vi "Agilent PSG MXG Series Digital Modulation.vi"() -> ()   [LabVIEW 2018]
doc: "This example shows how to configure the I/Q modulator and dual arbitrary waveform generator.\n\n<b>Notes:</b>\n(1) This VI is valid only in E8267C, E8267D, N5162A, N5182A, N5172B, N5182B.\n(2) For E8267C, this VI is valid only when the instrument installs <B>Option 002</B> (Internal baseband generator) or <B>Option 602</B> (Digital bus baseband generator).\n(3) For E8267D, this VI is valid only when the instrument installs <B>Option 601</B> or <B>Option 602</B> (Internal baseband generator).\n(4) For N5162A and N5182A, this VI is valid only when the instrument installs <B>Option 651</B> or <B>Option 652</B> or <B>Option 654</B> (Internal baseband generator)."
uses:
  Agilent PSG MXG Series.lvlib
panel:
  in  "I/Q Source (0: Ext 50 Ohms)":u16(ring) items=["Ext 50 Ohms", "Ext 600 Ohms", "Internal", "Baseband Generator", "Off", "Sum"]
  in  "VISA resource name":refnum<visa-resource-name>
  in  "Enable ARB (T:Enable)":bool=TRUE
  in  "External Q Offset (50 mV)":dbl=0.05
  in  "External I Offset (50 mV)":dbl=0.05
  in  "Differential Mode Q Offset (10 mV)":dbl=0.01
  in  "Differential Mode I Offset (10 mV)":dbl=0.01
  in  "Common Mode I/Q Offset (1 V)":dbl=1.0
  in  "Q Offset (10 percent)":dbl=10.0
  in  "I/Q Skew (0 s)":dbl
  in  "Quadrature Skew (5 deg)":dbl=5.0
  in  "Gain (0.5 dB)":dbl=0.5
  in  "I Offset (10 percent)":dbl=10.0
  in  "Enable I/Q Adjustment (F:Disable)":bool
  in  "I/Q Source No. (1)":u16(ring)=1 items=["1"=1, "2"=2]
  in  "I/Q Phase Polarity (0: Normal)":u16(ring) items=["Normal", "Inverted"]
  # "(c) 2007-2016 National Instruments.  ALL RIGHTS RESERVED."
  # "(1) This VI is valid only in E8267C, E8267D, N5162A, N5182A, N5172B, N5182B.\n(2) For E8267C, this VI is valid only when the instrument installs Option 002 or Option 602.\n(3) For E8267D, this VI is valid only when the instrument installs Option 601 or Option 602.\n(4) For N5162A and N5182A, this VI is valid only when the instrument installs Option 651 or Option 652 or Option 654."
  # "Note: Enable arbitrary\nwaveform generator."
  # "Note: These parameters are\nfor I/Q Adjustment."
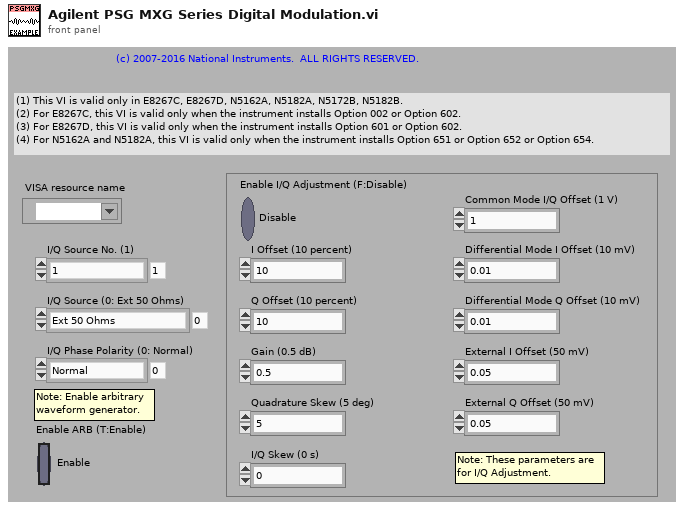
[diagram p1: front panel]
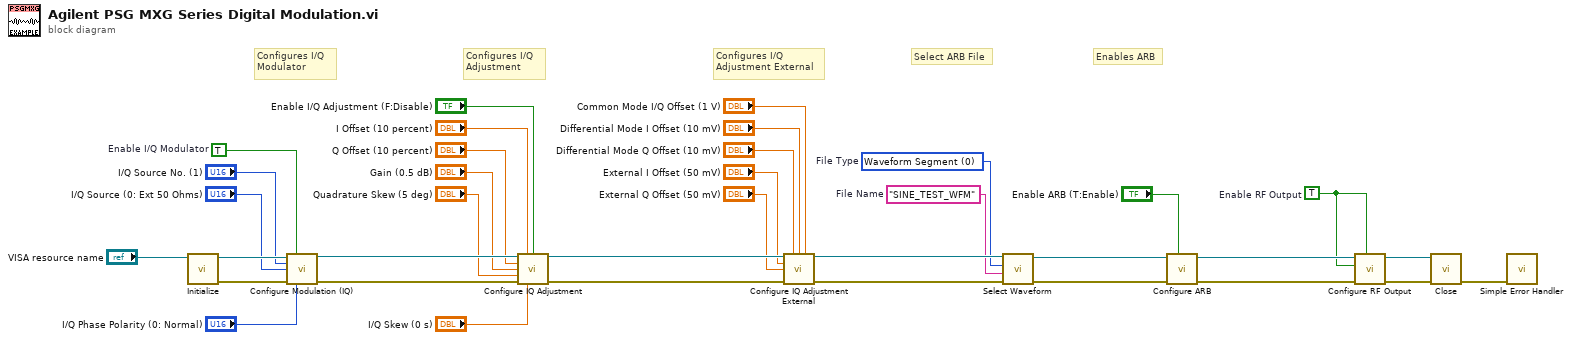
[diagram p0: block diagram]
diagram:
  w1 = TRUE  # Enable RF Output
  w11 = "SINE_TEST_WFM"  # File Name
  w12 = u16 0 items=["Waveform Segment", "Waveform Sequence"]  # File Type
  w33 = TRUE  # Enable I/Q Modulator
  # "Enables ARB"
  # "Select ARB File"
  # "Configures I/Q\nAdjustment External"
  # "Configures I/Q\nAdjustment"
  # "Configures I/Q\nModulator"
  n1 = call "Initialize.vi"("VISA resource name"="VISA resource name") -> ("error out"=w34:errorcluster, "VISA resource name out"=w35:refnum<visa-resource-name>)  [unwired: 3 in, 6 out]
  n2 = call "Configure Modulation (IQ).vi"("VISA resource name"=w35, "Enable I/Q Modulator (T:Enable)"=w33, "I/Q Source No. (1)"="I/Q Source No. (1)", "I/Q Source (0: Ext 50 Ohms)"="I/Q Source (0: Ext 50 Ohms)", "error in (no error)"=w34, "I/Q Phase Polarity (0: Normal)"="I/Q Phase Polarity (0: Normal)") -> ("VISA resource name out"=w30:refnum<visa-resource-name>, "error out"=w29:errorcluster)  [unwired: 4 in, 4 out]
  n3 = call "Configure IQ Adjustment.vi"("VISA resource name"=w30, "I Offset (0 percent)"="I Offset (10 percent)", "Enable I/Q Adjustment (F:Disable)"="Enable I/Q Adjustment (F:Disable)", "Q Offset (0 percent)"="Q Offset (10 percent)", "Gain (0 dB)"="Gain (0.5 dB)", "Quadrature Skew (0 deg)"="Quadrature Skew (5 deg)", "error in (no error)"=w29, "I/Q Skew (0 s)"="I/Q Skew (0 s)") -> ("VISA resource name out"=w22:refnum<visa-resource-name>, "error out"=w21:errorcluster)  [unwired: 2 in, 4 out]
  n4 = call "Configure IQ Adjustment External.vi"("VISA resource name"=w22, "Differential Mode Q Offset (0 V)"="Differential Mode Q Offset (10 mV)", "Differential Mode I Offset (0 V)"="Differential Mode I Offset (10 mV)", "Common Mode I/Q Offset (0 V)"="Common Mode I/Q Offset (1 V)", "External I Offset (0 V)"="External I Offset (50 mV)", "External Q Offset (0 V)"="External Q Offset (50 mV)", "error in (no error)"=w21) -> ("VISA resource name out"=w14:refnum<visa-resource-name>, "error out"=w13:errorcluster)  [unwired: 3 in, 4 out]
  n5 = call "Select Waveform.vi"("error in (no error)"=w13, "File Name (\"\")"=w11, "File Type (0: Waveform Segment)"=w12, "VISA resource name"=w14) -> ("error out"=w9:errorcluster, "VISA resource name out"=w10:refnum<visa-resource-name>)  [unwired: 6 out]
  n6 = call "Configure ARB.vi"("Enable ARB (T:Enable)"="Enable ARB (T:Enable)", "error in (no error)"=w9, "VISA resource name"=w10) -> ("error out"=w4:errorcluster, "VISA resource name out"=w5:refnum<visa-resource-name>)  [unwired: 1 in, 6 out]
  n7 = call "Configure RF Output.vi"("Enable Modulation (T:Enable)"=w1, "error in (no error)"=w4, "Enable RF Output (F:Disable)"=w1, "VISA resource name"=w5) -> ("error out"=w2:errorcluster, "VISA resource name out"=w3:refnum<visa-resource-name>)  [unwired: 3 in, 3 out]
  n8 = call "Close.vi"("error in (no error)"=w2, "VISA resource name"=w3) -> ("error out"=w15:errorcluster)  [unwired: 9 out]
  n9 = call <vilib>:"Simple Error Handler.vi"("error in (no error)"=w15) -> ()  [unwired: 1 in, 8 out]
